vi "navX Open.vi"(5 "I2C Bus":T6=enum."I2C MXP", 7 "SPI Bus":T4=enum."SPI MXP", 8 "error in":errorcluster, 10 "Update Rate (4Hz-60Hz)":T13=50 min=4 max=50 step=1, 11 "navX Interface Protocol":T2) -> (0 "error out":errorcluster, 1 "Opened?":bool, 3 "navX Device TypeDef":T1={"navX Interface Protocol"=enum."SPI", "navX Interface Protocol TypeDefs"={"SPIDevRef"={"DevStatus"={"status"=FALSE, "code"=0, "source"=""}, "Handle"=0, "SPI Bus"=enum."SPI On-Board, CS0"}, "I2CDevRef"={"DevStatus"={"status"=FALSE, "code"=0, "source"=""}, "Device Address"=0, "Handle"=0, "I2C Bus"=enum."Invalid"}}, "navX System Information"={"Board Information"={"WhoAmI (50 | 0x32)"=0, "Board Revision"=0, "Firmware Major Version"=0, "Firmware Minor Version"=0}, "Status"={"Update Rate Hz"=0, "Accelerometer Full-Scale Range"=0, "Gyro Full-Scale Range"=0, "NAVX_OP_STATUS"=0, "NAVX_CAL_STATUS"=0, "NAVX_SELFTEST_STATUS"=0, "NAVX_SENSOR_STATUS"={"MOVING"=FALSE, "YAW_STABLE"=FALSE, "MAG_DISTURBANCE"=FALSE, "ALTITUDE_VALID"=FALSE, "SEALEVEL_PRESS_SET"=FALSE, "FUSED_HEADING_VALID"=FALSE}}, "Offsets"={"Yaw"=0.0, "Quat W"=0.0, "Quat X"=0.0, "Quat Y"=0.0, "Quat Z"=0.0}}, "navX Common Information"={"Update Rate (4Hz-60Hz)"=50, "refnum name"="", "error"={"status"=FALSE, "code"=0, "source"=""}}} {"navX Common Information"."Update Rate (4Hz-60Hz)" min=4 max=50 step=1; "navX System Information"."Status"."NAVX_OP_STATUS" items=["INITIALIZING", "SELFTEST_IN_PROGRESS", "ERROR", "IMU_AUTOCAL_IN_PROGRESS", "NORMAL"]; "navX System Information"."Status"."NAVX_CAL_STATUS" items=["IMU_CAL_STATE_MASK"=3, "IMU_CAL_INPROGRESS"=0, "IMU_CAL_ACCUMULATE"=1, "IMU_CAL_COMPLETE"=2, "MAG_CAL_COMPLETE"=4, "BARO_CAL_COMPLETE"=8]; "navX Interface Protocol TypeDefs"."I2CDevRef"."Device Address" format="%.0x"})   [LabVIEW 2015, in "navX-MXP IMU.lvlib"]
uses:
  navX-MXP IMU.lvlib
  TypeDefs/Value TypeDefs/navX Interface Protocol.ctl
  TypeDefs/Value TypeDefs/navX Update Rate.ctl
  <vilib>/Rock Robotics/SystemInterfaces/spilib/spi_bus.ctl
  <vilib>/Rock Robotics/SystemInterfaces/i2clib/i2c_bus.ctl
  TypeDefs/navX Device TypeDef.ctl
  <vilib>/Rock Robotics/WPI/SPI/WPI_SPIDevRef.ctl
  <vilib>/Rock Robotics/WPI/I2C/WPI_I2CDevRef.ctl
  TypeDefs/Data TypeDefs/navX Board Information.ctl
  TypeDefs/Data TypeDefs/navX Status Data.ctl
  TypeDefs/Value TypeDefs/navX NAVX_OP_STATUS.ctl
  TypeDefs/Value TypeDefs/navX NAVX_CAL_STATUS.ctl
  TypeDefs/Value TypeDefs/navX NAVX_SENSOR_STATUS.ctl
  TypeDefs/Data TypeDefs/navX Offsets Data.ctl
  TypeDefs/Value TypeDefs/navX Device Registers.ctl
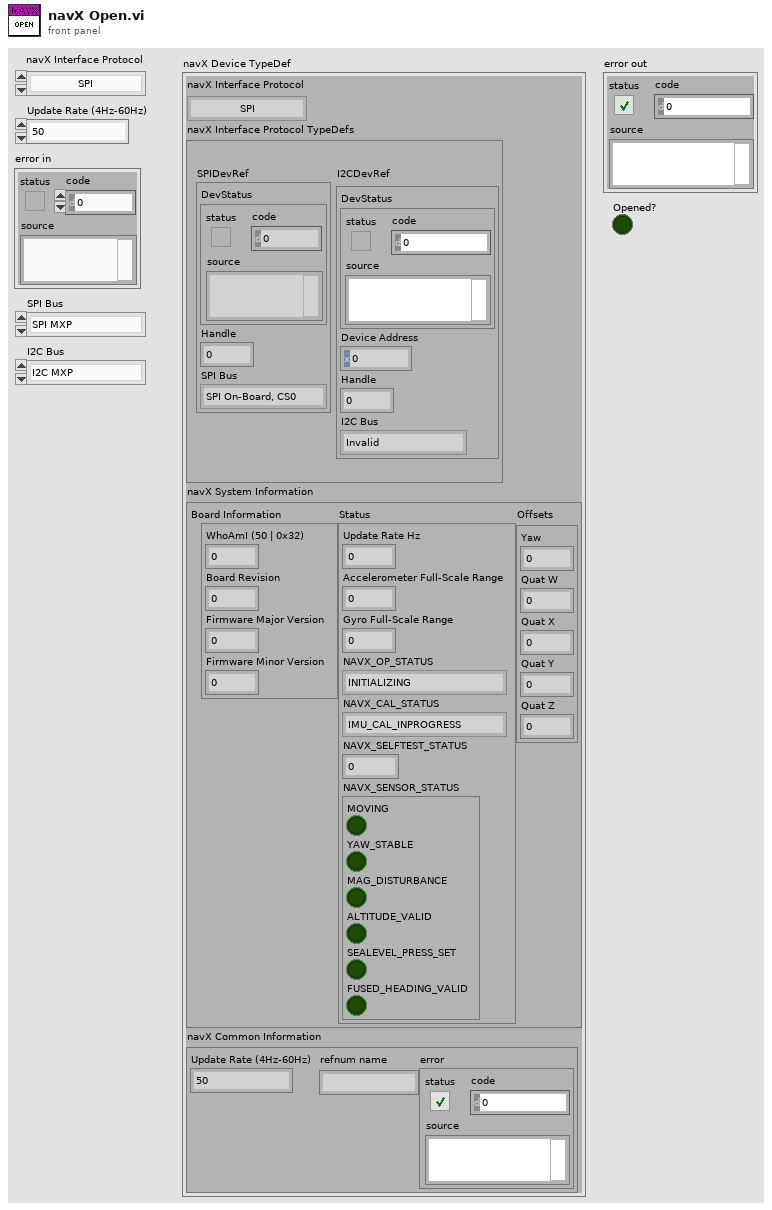
[diagram p1: front panel]
types:
  T1 = typedef "navX-MXP IMU.lvlib/navX Device TypeDef.ctl" = cluster{"navX Interface Protocol":T2, "navX Interface Protocol TypeDefs":cluster{"SPIDevRef":T3, "I2CDevRef":T5}, "navX System Information":cluster{"Board Information":T7, "Status":T8, "Offsets":T12}, "navX Common Information":cluster{"Update Rate (4Hz-60Hz)":T13, "refnum name":string, "error":errorcluster}}
  T2 = typedef "navX-MXP IMU.lvlib/navX Interface Protocol.ctl" = enum16{"SPI", "I2C"}
  T3 = typedef "WPI_SPIDevRef.ctl" = cluster{"DevStatus":errorcluster, "Handle":i32, "SPI Bus":T4}
  T4 = typedef "spi_bus.ctl" = enum16{"SPI On-Board, CS0", "SPI On-Board, CS1", "SPI On-Board, CS2", "SPI On-Board, CS3", "SPI MXP", "Invalid"}
  T5 = typedef "WPI_I2CDevRef.ctl" = cluster{"DevStatus":errorcluster, "Device Address":u8, "Handle":i32, "I2C Bus":T6}
  T6 = typedef "i2c_bus.ctl" = enum16{"I2C On-Board", "I2C MXP", "Invalid"}
  T7 = typedef "navX-MXP IMU.lvlib/navX Board Information.ctl" = cluster{"WhoAmI (50 | 0x32)":u8, "Board Revision":u8, "Firmware Major Version":u8, "Firmware Minor Version":u8}
  T8 = typedef "navX-MXP IMU.lvlib/navX Status Data.ctl" = cluster{"Update Rate Hz":u8, "Accelerometer Full-Scale Range":u8, "Gyro Full-Scale Range":u16, "NAVX_OP_STATUS":T9, "NAVX_CAL_STATUS":T10, "NAVX_SELFTEST_STATUS":u8, "NAVX_SENSOR_STATUS":T11}
  T9 = typedef "navX-MXP IMU.lvlib/navX NAVX_OP_STATUS.ctl" = u8
  T10 = typedef "navX-MXP IMU.lvlib/navX NAVX_CAL_STATUS.ctl" = u8
  T11 = typedef "navX-MXP IMU.lvlib/navX NAVX_SENSOR_STATUS.ctl" = cluster{"MOVING":bool, "YAW_STABLE":bool, "MAG_DISTURBANCE":bool, "ALTITUDE_VALID":bool, "SEALEVEL_PRESS_SET":bool, "FUSED_HEADING_VALID":bool}
  T12 = typedef "navX-MXP IMU.lvlib/navX Offsets Data.ctl" = cluster{"Yaw":dbl, "Quat W":dbl, "Quat X":dbl, "Quat Y":dbl, "Quat Z":dbl}
  T13 = typedef "navX-MXP IMU.lvlib/navX Update Rate.ctl" = u8
  T14 = typedef "navX-MXP IMU.lvlib/navX Device Registers.ctl" = u8
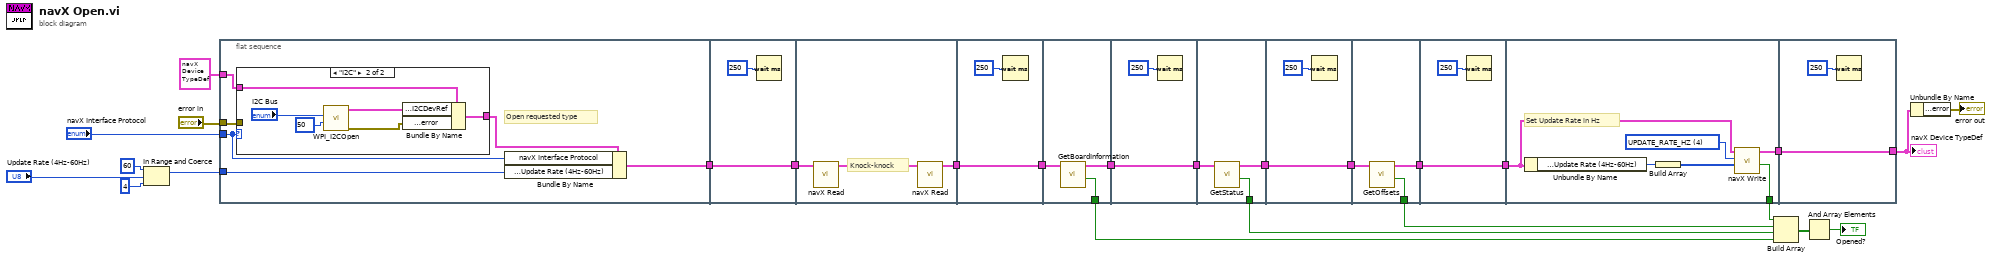
[diagram p0: block diagram]
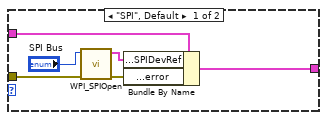
[diagram p2: hidden frame]
diagram:
  n1 = In Range and Coerce(upper limit=u8 60, x="Update Rate (4Hz-60Hz)", lower limit=u8 4) -> (coerced(x)=w14:T13)  [unwired: 1 out]
  n2 = flat-sequence {
    tunnel: "navX Interface Protocol" -> [w32]
    tunnel: T1 {"navX Interface Protocol"=enum."SPI", "navX Interface Protocol TypeDefs"={"SPIDevRef"={"DevStatus"={"status"=FALSE, "code"=0, "source"=""}, "Handle"=0, "SPI Bus"=enum."SPI On-Board, CS0"}, "I2CDevRef"={"DevStatus"={"status"=FALSE, "code"=0, "source"=""}, "Device Address"=0, "Handle"=0, "I2C Bus"=enum."Invalid"}}, "navX System Information"={"Board Information"={"WhoAmI (50 | 0x32)"=0, "Board Revision"=0, "Firmware Major Version"=0, "Firmware Minor Version"=0}, "Status"={"Update Rate Hz"=0, "Accelerometer Full-Scale Range"=0, "Gyro Full-Scale Range"=0, "NAVX_OP_STATUS"=0, "NAVX_CAL_STATUS"=0, "NAVX_SELFTEST_STATUS"=0, "NAVX_SENSOR_STATUS"={"MOVING"=FALSE, "YAW_STABLE"=FALSE, "MAG_DISTURBANCE"=FALSE, "ALTITUDE_VALID"=FALSE, "SEALEVEL_PRESS_SET"=FALSE, "FUSED_HEADING_VALID"=FALSE}}, "Offsets"={"Yaw"=0.0, "Quat W"=0.0, "Quat X"=0.0, "Quat Y"=0.0, "Quat Z"=0.0}}, "navX Common Information"={"Update Rate (4Hz-60Hz)"=50, "refnum name"="", "error"={"status"=FALSE, "code"=0, "source"=""}}} ("navX Device TypeDef") -> [w31]
    tunnel: "error in" -> [w29]
    tunnel: w14 -> [w27]
    tunnel: [w28] -> w19
    tunnel: w19 -> [w46]
    tunnel: [w46] -> w18
    tunnel: w18 -> [w49]
    tunnel: [w47] -> w20
    tunnel: w20 -> [w50]
    tunnel: [w50] -> w21
    tunnel: w21 -> [w53]
    tunnel: [w54] -> w3
    tunnel: [w52] -> w11
    tunnel: w3 -> [w56]
    tunnel: [w56] -> w2
    tunnel: w2 -> [w58]
    tunnel: [w59] -> w5
    tunnel: [w57] -> w10
    tunnel: w5 -> [w61]
    tunnel: [w61] -> w4
    tunnel: w4 -> [w63]
    tunnel: [w62] -> w9
    tunnel: [w64] -> w7
    tunnel: w7 -> [w66]
    tunnel: [w66] -> w6
    tunnel: [w67] -> w8
    tunnel: w6 -> [w69]
    tunnel: [w68] -> w1
    tunnel: [w74] -> w23
    tunnel: w1 -> [w74]
    frame #0 {
      # "Open requested type"
      n3 = case shown="\"I2C\"" w32 {
        tunnel: w31 -> [w38 w44]
        tunnel: [w35 w43] -> w30
        tunnel: w29 -> [w34 _]
        frame "SPI", Default {
          n4 = call <vilib>:"WPI_SPIOpen.vi"("error in"=w34, "SPI Bus"="SPI Bus") -> ("error out"=w37:errorcluster, "SPIDevRef"=w36:T3)  [unwired: 8 in]
          n5 = Bundle By Name(cluster=w38, "navX Interface Protocol TypeDefs.SPIDevRef"=w36, "navX Common Information.error"=w37) -> (w35:T1)
        }
        frame "I2C" {
          n6 = call <vilib>:"WPI_I2COpen.vi"("Device Address"=u8 50, "I2C Bus"="I2C Bus") -> ("error out"=w42:errorcluster, "I2CDevRef"=w41:T5)  [unwired: 8 in]
          n7 = Bundle By Name(cluster=w44, "navX Interface Protocol TypeDefs.I2CDevRef"=w41, "navX Common Information.error"=w42) -> (w43:T1)
        }
      }
      n8 = Bundle By Name(cluster=w30, "navX Interface Protocol"=w32, "navX Common Information.Update Rate (4Hz-60Hz)"=w27) -> (w28:T1)
    }
    frame #1 {
      n9 = Wait (ms)(milliseconds to wait=u32 250) -> ()  [unwired: 1 out]
    }
    frame #2 {
      # "Knock-knock"
      n10 = call "navX Read.vi"("navX Device TypeDef"=w49) -> ("navX Device TypeDef"=w48:T1)  [unwired: 8 in, 2 out]
      n11 = call "navX Read.vi"("navX Device TypeDef"=w48) -> ("navX Device TypeDef"=w47:T1)  [unwired: 8 in, 2 out]
    }
    frame #3 {
      n12 = Wait (ms)(milliseconds to wait=u32 250) -> ()  [unwired: 1 out]
    }
    frame #4 {
      n13 = call "GetBoardInformation.vi"("navX Device TypeDef"=w53) -> ("Valid?"=w52:bool, "navX Device TypeDef"=w54:T1)  [unwired: 8 in, 1 out]
    }
    frame #5 {
      n14 = Wait (ms)(milliseconds to wait=u32 250) -> ()  [unwired: 1 out]
    }
    frame #6 {
      n15 = call "GetStatus.vi"("navX Device TypeDef"=w58) -> ("Valid?"=w57:bool, "navX Device TypeDef"=w59:T1)  [unwired: 8 in, 1 out]
    }
    frame #7 {
      n16 = Wait (ms)(milliseconds to wait=u32 250) -> ()  [unwired: 1 out]
    }
    frame #8 {
      n17 = call "GetOffsets.vi"("navX Device TypeDef"=w63) -> ("Valid?"=w62:bool, "navX Device TypeDef"=w64:T1)  [unwired: 8 in, 1 out]
    }
    frame #9 {
      n18 = Wait (ms)(milliseconds to wait=u32 250) -> ()  [unwired: 1 out]
    }
    frame #10 {
      w72 = T14 4 items=["WHOAMI"=0, "HW_REV"=1, "FW_VER_MAJOR"=2, "FW_VER_MINOR"=3, "UPDATE_RATE_HZ"=4, "ACCEL_FSR_G"=5, "GYRO_FSR_DPS"=6, "OP_STATUS"=8, "CAL_STATUS"=9, "SELFTEST_STATUS"=10, "SENSOR_STATUS"=16, "TIMESTAMP"=18, "YAW"=22, "PITCH"=24, "ROLL"=26, "HEADING"=28, "FUSED_HEADING"=30, "ALTITUDE_I"=32, "ALTITUDE_D"=34, "LINERA_ACC_X"=36, "LINERA_ACC_Y"=38, "LINERA_ACC_Z"=40, "QUAT_W"=42, "QUAT_X"=44, "QUAT_Y"=46, "QUAT_Z"=48, "MPU_TEMP_C"=50, "GYRO_X"=52, "GYRO_Y"=54, "GYRO_Z"=56, "ACC_X"=58, "ACC_Y"=60, "ACC_Z"=62, "MAG_X"=64, "MAG_Y"=66, "MAG_Z"=68, "PRESSURE_I"=70, "PRESSURE_D"=72, "PRESSURE_TEMP"=74, "YAW_OFFSET"=76, "QUAT_OFFSET_W"=78, "QUAT_OFFSET_X"=80, "QUAT_OFFSET_Y"=82, "QUAT_OFFSET_Z"=84] ("Device Register")
      # "Set Update Rate in Hz"
      n19 = Unbundle By Name(w69) -> ("navX Common Information.Update Rate (4Hz-60Hz)"=w71:T13)
      n20 = Build Array(w71) -> (w70:T13[])
      n21 = call "navX Write.vi"("navX Message"=w70, "Device Register"=w72, "navX Device TypeDef"=w69) -> ("Valid?"=w67:bool, "navX Device TypeDef"=w68:T1)  [unwired: 7 in]
    }
    frame #11 {
      n22 = Wait (ms)(milliseconds to wait=u32 250) -> ()  [unwired: 1 out]
    }
  }
  n23 = Build Array(w8, w9, w10, w11) -> (w13:bool[])
  n24 = And Array Elements(Boolean array=w13) -> (logical AND=→"Opened?":bool)
  n25 = Unbundle By Name(w23) -> ("navX Common Information.error"=→"error out":errorcluster)
  "navX Device TypeDef" <- w23
